vi "Abort.vi"(8 "error in (no error)":errorcluster, 11 "VISA resource name":refnum<visa-resource-name>) -> (0 "error out":errorcluster, 3 "VISA resource name out":refnum<visa-resource-name>)   [LabVIEW 2019, in "Stanford Research 830.lvlib"]
doc: "Reset the scan.\n\n<B>Note:</B>\n\nAll stored data will be lost after executing this VI."
uses:
  Stanford Research 830.lvlib
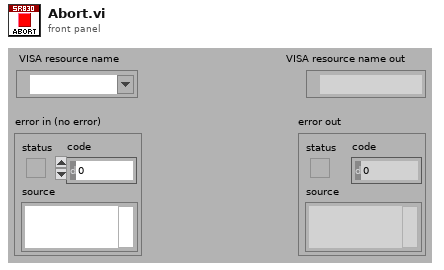
[diagram p1: front panel]
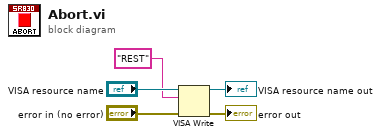
[diagram p0: block diagram]
diagram:
  n1 = VISA Write(VISA resource name="VISA resource name", write buffer="REST", error in (no error)="error in (no error)") -> (VISA resource name out=→"VISA resource name out":refnum<visa-resource-name>, error out=→"error out":errorcluster)  [unwired: 1 out]
